vi "Motor_Controller.vi"(4 "Friction Compensation(F)":bool, 6 "Reinitialize? (F)":bool, 8 "error in (no error)":errorcluster, 9 "Mode":T1, 10 "CableTensionRef(N)":dbl[](array[numeric]), 11 "Motor in":refnum<class "MotorControl.lvclass">) -> (0 "error out":errorcluster, 2 "VoltageCommand":dbl[](array[numeric]) format="%.2f", 3 "Motor out":refnum<class "MotorControl.lvclass">)   [LabVIEW 2015, in "MotorControl.lvclass"]
uses:
  MotorControl.lvclass
  TypeDef/MotorMode.ctl
  MotorControl.lvclass/MotorControl.ctl
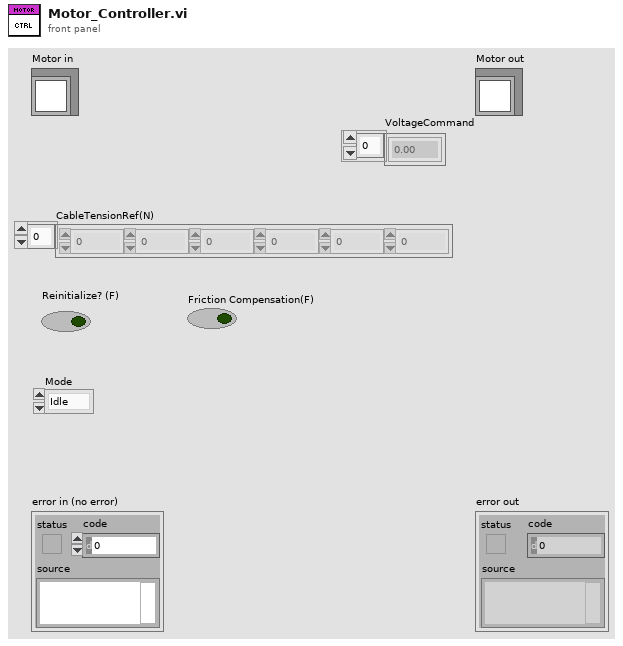
[diagram p1: front panel]
types:
  T1 = typedef "MotorControl.lvclass/MotorMode.ctl" = enum16{"Idle", "FF", "PID"}
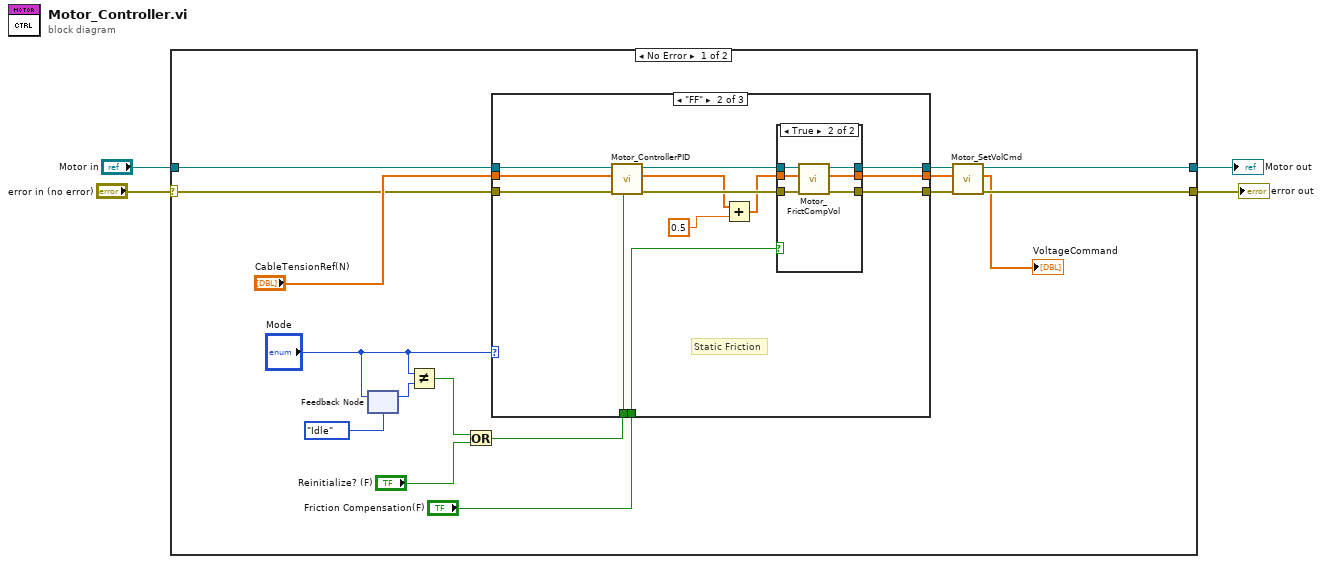
[diagram p0: block diagram]
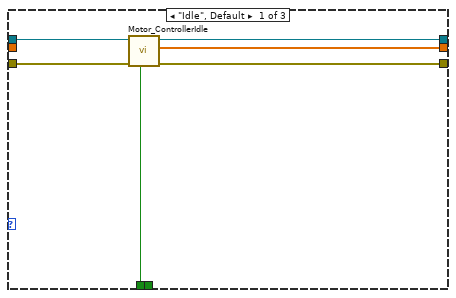
[diagram p2: hidden frame]
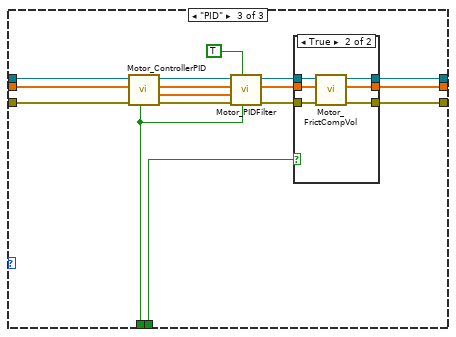
[diagram p4: hidden frame]
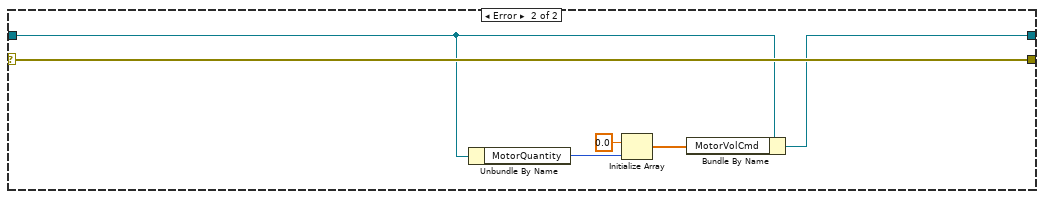
[diagram p6: hidden frame]
diagram:
  n1 = case shown="No Error" "error in (no error)" {
    selector: "error in (no error)" -> [w19 w79]
    tunnel: [w7 w79] -> w3
    tunnel: [w9 w74] -> w1
    tunnel: "Motor in" -> [w18 w75]
    frame No Error {
      n2 = feedback-in #1("Mode") -> ()
      n3 = feedback #1(MotorMode."Idle" ("Mode")) -> (w16:T1)
      n4 = Not Equal?(x="Mode", y=w16) -> (x != y?=w14:bool)
      n5 = Or(x=w14, y="Reinitialize? (F)") -> (x .or. y?=w12:bool)
      n6 = case shown="\"FF\"" "Mode" {
        tunnel: "CableTensionRef(N)" -> [_ w37 w62]
        tunnel: w19 -> [w26 w39 w64]
        tunnel: w18 -> [w25 w38 w63]
        tunnel: w12 -> [w22 w31 w52]
        tunnel: [w23 w35 w56] -> w8
        tunnel: [w24 w36 w57] -> w10
        tunnel: [w21 w33 w49] -> w6
        tunnel: "Friction Compensation(F)" -> [_ w34 w51]
        frame "Idle", Default {
          n7 = call "Motor_ControllerIdle.vi"("Reinitialize"=w22, "error in (no error)"=w26, "Motor Control in"=w25) -> ("error out"=w23:errorcluster, "VoltageCommand"=w21:dbl[], "Motor Control out"=w24:refnum<class "MotorControl.lvclass">)  [unwired: 6 in]
        }
        frame "FF" {
          # "Static Friction"
          n8 = call "Motor_ControllerPID.vi"("Reinitialize? (F)"=w31, "error in (no error)"=w39, "CableTensionRef(N)"=w37, "Motor in"=w38) -> ("error out"=w30:errorcluster, "FF cmd"=w29:dbl[], "Motor out"=w32:refnum<class "MotorControl.lvclass">)  [unwired: 2 in, 3 out]
          n9 = Add(x=w29, y=0.5 ("Numeric")) -> (x+y=w28:dbl[])
          n10 = case shown="True" w34 {
            tunnel: w30 -> [w41 w48]
            tunnel: w32 -> [w42 w47]
            tunnel: [w42 w46] -> w36
            tunnel: [w41 w45] -> w35
            tunnel: w28 -> [w40 w44]
            tunnel: [w40 w43] -> w33
            frame False {
            }
            frame True {
              n11 = call-dynamic "Motor_FrictCompVol.vi"("error in (no error)"=w48, "Input Vol"=w44, "Motor in"=w47) -> ("error out"=w45:errorcluster, "Fric Vol + Input Vol"=w43:dbl[], "Motor out"=w46:refnum<class "MotorControl.lvclass">)  [unwired: 5 in, 1 out]
            }
          }
        }
        frame "PID" {
          n12 = call "Motor_ControllerPID.vi"("Reinitialize? (F)"=w52, "error in (no error)"=w64, "CableTensionRef(N)"=w62, "Motor in"=w63) -> ("error out"=w58:errorcluster, "PID cmd"=w55:dbl[], "FF cmd"=w54:dbl[], "Motor out"=w59:refnum<class "MotorControl.lvclass">)  [unwired: 2 in, 2 out]
          n13 = call "Motor_PIDFilter.vi"("Initialize (F)"=w52, "Softload? (T)"=TRUE, "error in (no error)"=w58, "PID cmd in"=w55, "FF cmd in"=w54, "Motors_New in"=w59) -> ("error out"=w61:errorcluster, "Filtered PID + FF"=w50:dbl[], "Motors_New out"=w60:refnum<class "MotorControl.lvclass">)  [unwired: 2 in, 1 out]
          n14 = case shown="True" w51 {
            tunnel: w61 -> [w66 w73]
            tunnel: w60 -> [w67 w72]
            tunnel: [w67 w71] -> w57
            tunnel: [w66 w70] -> w56
            tunnel: w50 -> [w65 w69]
            tunnel: [w65 w68] -> w49
            frame False {
            }
            frame True {
              n15 = call-dynamic "Motor_FrictCompVol.vi"("error in (no error)"=w73, "Input Vol"=w69, "Motor in"=w72) -> ("error out"=w70:errorcluster, "Fric Vol + Input Vol"=w68:dbl[], "Motor out"=w71:refnum<class "MotorControl.lvclass">)  [unwired: 5 in, 1 out]
            }
          }
        }
      }
      n16 = call "Motor_SetVolCmd.vi"("error in (no error)"=w8, "VolCmd"=w6, "MotorCtrl in"=w10) -> ("error out"=w7:errorcluster, "VolCmdOutput"=→"VoltageCommand":dbl[], "MotorCtrl out"=w9:refnum<class "MotorControl.lvclass">)  [unwired: 6 in]
    }
    frame Error {
      n17 = Unbundle By Name(w75) -> ("MotorQuantity"=w78:i32)
      n18 = Initialize Array(0.0 ("element"), w78) -> (w76:dbl[])
      n19 = Bundle By Name(cluster=w75, "MotorVolCmd"=w76) -> (w74:refnum<class "MotorControl.lvclass">)
    }
  }
  "error out" <- w3
  "Motor out" <- w1
